vi "GUIReader.vi"(2 "Input Array":dbl[](array[numeric])) -> (0 "hinten LI":dbl, 1 "Links":dbl, 3 "Hinten R":dbl, 4 "Rechts":dbl, 5 "Linefollow_Array":bool[](array[boolean]), 6 "Schräg L":dbl, 7 "gerade L":dbl, 9 "gerade R":dbl, 10 "Schräg R":dbl)   [LabVIEW 2016]
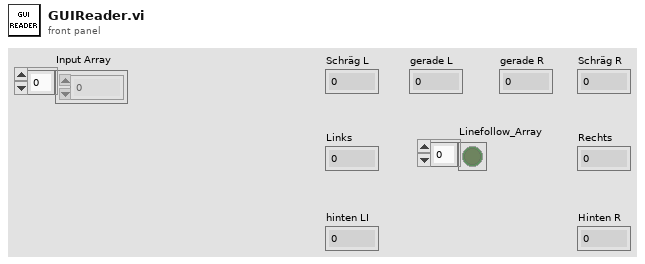
[diagram p1: front panel]
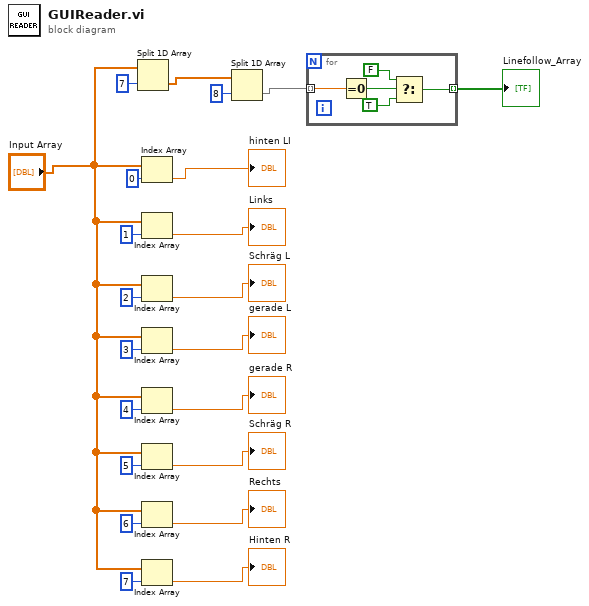
[diagram p0: block diagram]
diagram:
  n1 = Split 1D Array(array="Input Array", index=7) -> (second subarray=w4:dbl[])  [unwired: 1 out]
  n2 = Index Array(array="Input Array", index=0) -> (element=→"hinten LI":dbl)
  n3 = Index Array(array="Input Array", index=1) -> (element=→"Links":dbl)
  n4 = Index Array(array="Input Array", index=2) -> (element=→"Schräg L":dbl)
  n5 = Index Array(array="Input Array", index=3) -> (element=→"gerade L":dbl)
  n6 = Index Array(array="Input Array", index=4) -> (element=→"gerade R":dbl)
  n7 = Index Array(array="Input Array", index=5) -> (element=→"Schräg R":dbl)
  n8 = Index Array(array="Input Array", index=6) -> (element=→"Rechts":dbl)
  n9 = Index Array(array="Input Array", index=7) -> (element=→"Hinten R":dbl)
  n10 = Split 1D Array(array=w4, index=8) -> (second subarray=w2:dbl[])  [unwired: 1 out]
  n11 = for {
    tunnel: w2 -> [w27] mode=indexing
    tunnel: [w23] -> w1 mode=indexing
    n12 = Equal To 0?(x=w27) -> (x = 0?=w26:bool)
    n13 = Select(t=FALSE, s=w26, f=TRUE) -> (s? t:f=w23:bool)
  }
  "Linefollow_Array" <- w1
